vi "Write.vi"(9 "Data":u8 format="%02x", 10 "Address":u16 format="%04x", 11 "EEPROM in":refnum<class "RAM.lvclass">) -> (3 "EEPROM out":refnum<class "RAM.lvclass">)   [LabVIEW 2021, in "RAM.lvclass"]
uses:
  RAM.lvclass
  RAM.lvclass/RAM.ctl
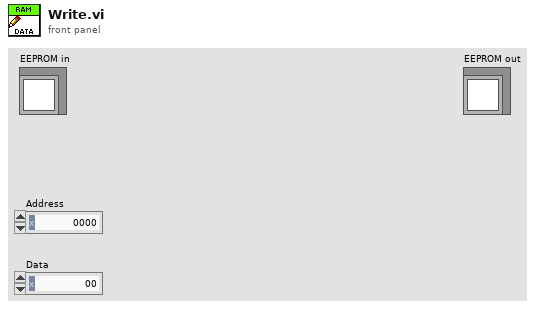
[diagram p1: front panel]
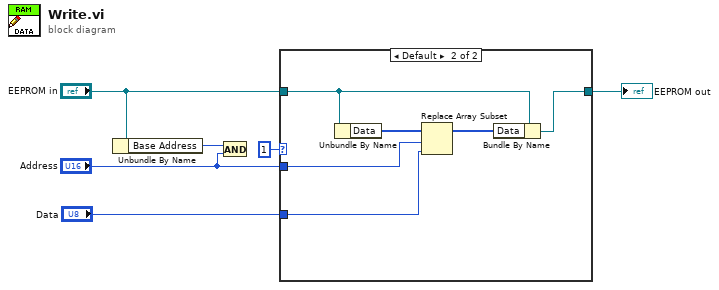
[diagram p0: block diagram]
diagram:
  n1 = Unbundle By Name("EEPROM in") -> ("Base Address"=w3:u16)
  n2 = And(x=w3, y="Address") -> ()  [unwired: 1 out]
  n3 = case shown="Default" u16 1 {
    tunnel: "EEPROM in" -> [w7 w10]
    tunnel: [w7 w12] -> w5
    tunnel: "Data" -> [_ w11]
    tunnel: "Address" -> [_ w8]
    frame 0 {
    }
    frame Default {
      n4 = Unbundle By Name(w10) -> ("Data"=w9:u8[])
      n5 = Replace Array Subset(array=w9, new element=w11, index=w8) -> (w13:u8[])
      n6 = Bundle By Name(cluster=w10, "Data"=w13) -> (w12:refnum<class "RAM.lvclass">)
    }
  }
  "EEPROM out" <- w5
